vi "Dashboard Loop.vi"(7 "connection ID":refnum<k16>) -> ()   [LabVIEW 2014]
uses:
  Common Code/Dashboard Display Data.ctl
  Robot Global Data.vi
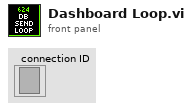
[diagram p1: front panel]
types:
  T1 = typedef "Dashboard Display Data.ctl" = cluster{"Gyro Angle":dbl}
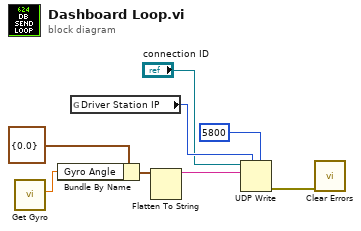
[diagram p0: block diagram]
diagram:
  n1 = call "Get Gyro.vi"() -> ("Angle"=w7:dbl)  [unwired: 11 in]
  n2 = Bundle By Name(cluster=T1 {"Gyro Angle"=0.0} ("Cluster"), "Gyro Angle"=w7) -> (w6:T1)
  n3 = global read "Robot Global Data.vi" "Driver Station IP"() -> (w4:u32)
  n4 = Flatten To String(anything=w6) -> (data string=w5:string)  [unwired: 3 in, 2 out]
  n5 = UDP Write(address=w4, port or service name=u16 5800, connection ID="connection ID", data in=w5) -> (error out=w3:errorcluster)  [unwired: 2 in, 1 out]
  n6 = call <vilib>:"Clear Errors.vi"("error in (no error)"=w3) -> ()  [unwired: 5 in, 2 out]
